vi "01_AMT_EEROM.vi"(2 "Number":u32, 3 "Command":enum16{"Init", "EERD", "EEWR"}(ring)) -> (1 "Response":string)   [LabVIEW 2020]
panel:
  in  "Memory":u8[](array[numeric]) format="%.0x"
  out "Array":u16[](array[numeric]) format="%.0x"
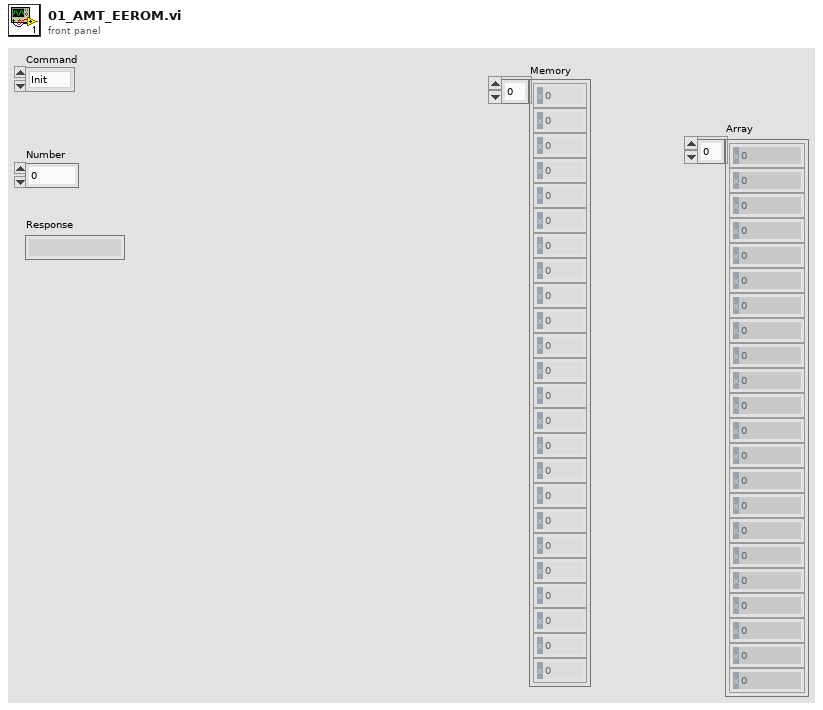
[diagram p1: front panel]
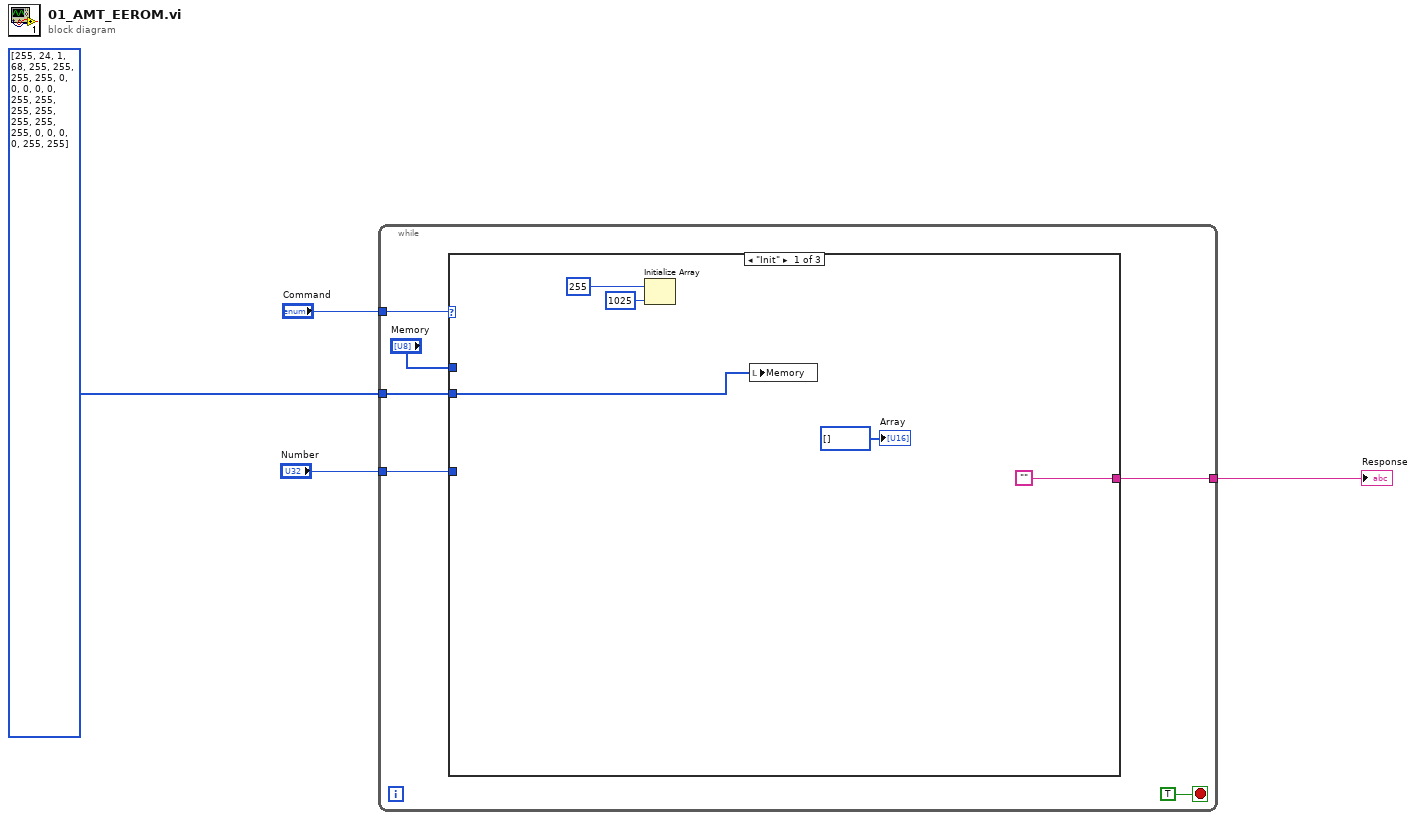
[diagram p0: block diagram]
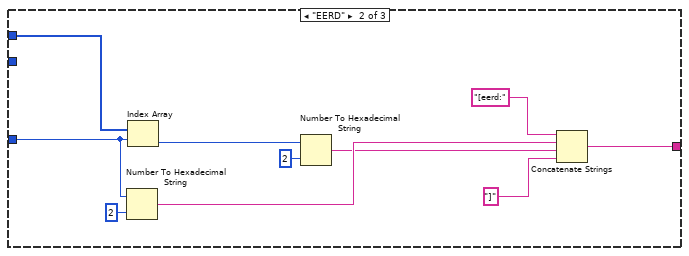
[diagram p2: hidden frame]
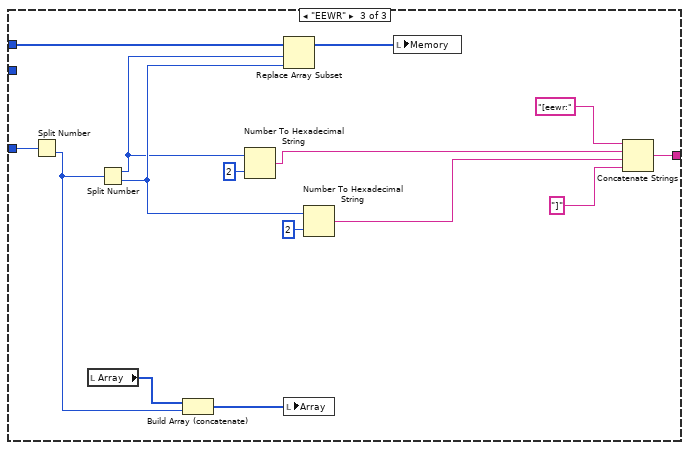
[diagram p3: hidden frame]
diagram:
  n1 = while {
    tunnel: "Command" -> [w10]
    tunnel: "Number" -> [w8]
    tunnel: [w7] -> w2
    tunnel: u8[] [255, 24, 1, 68, 255, 255, 255, 255, 0, 0, 0, 0, 0, 255, 255, 255, 255, 255, 255, 255, 0, 0, 0, 0, 255, 255] ("initialized array") -> [w5]
    stop <- TRUE stop-if-true
    n2 = case shown="\"Init\"" w10 {
      tunnel: "Memory" -> [_ w16 w36]
      tunnel: w8 -> [_ w25 w38]
      tunnel: ["" w21 w27] -> w7
      tunnel: w5 -> [w11 _ _]
      frame "Init" {
        n3 = Initialize Array(u8 255, 1025 ("dimension size")) -> ()  [unwired: 1 out]
        n4 = local write "Memory"(w11) -> ()
        "Array" <- u8[] [] ("Array")
      }
      frame "EERD" {
        n5 = Number To Hexadecimal String(1:i16 2 ("width (-)"), 2:w25) -> (0:w18:string)
        n6 = Index Array(array=w16, index=w25) -> (element=w22:u8)
        n7 = Number To Hexadecimal String(1:i16 2 ("width (-)"), 2:w22) -> (0:w17:string)
        n8 = Concatenate Strings("[eerd:" ("string"), w18, w17, "]" ("string")) -> (w21:string)
      }
      frame "EEWR" {
        n9 = Split Number(x=w38) -> (lo(x)=w37:u16)  [unwired: 1 out]
        n10 = local read "Array"() -> (w40:u16[])
        n11 = Split Number(x=w37) -> (hi(x)=w32:u8, lo(x)=w34:u8)
        n12 = Build Array (concatenate)(w40, w37) -> (w39:u16[])
        n13 = Number To Hexadecimal String(1:i16 2 ("width (-)"), 2:w32) -> (0:w29:string)
        n14 = Replace Array Subset(array=w36, new element=w34, index=w32) -> (w26:u8[])
        n15 = local write "Array"(w39) -> ()
        n16 = Number To Hexadecimal String(1:i16 2 ("width (-)"), 2:w34) -> (0:w28:string)
        n17 = local write "Memory"(w26) -> ()
        n18 = Concatenate Strings("[eewr:" ("string"), w29, w28, "]" ("string")) -> (w27:string)
      }
    }
  }
  "Response" <- w2
